vi "get action name.vi"(11 "action in":refnum<class "action.lvclass">) -> (2 "action name":string, 3 "action out":refnum<class "action.lvclass">)   [LabVIEW 2013, in "action.lvclass"]
uses:
  action.lvclass
  action.lvclass/action.ctl
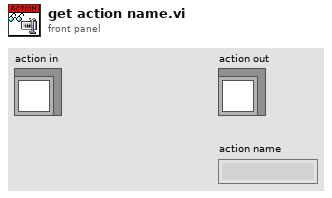
[diagram p1: front panel]
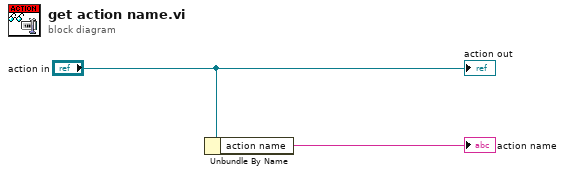
[diagram p0: block diagram]
diagram:
  n1 = Unbundle By Name("action in") -> ("action name"=→"action name":string)
  "action out" <- "action in"
